vi "frontp_unregister_UI_user_events.vi"(8 "error in (no error)":errorcluster, 11 "front_panel in":refnum<class "front_panel.lvclass">) -> (0 "error out":errorcluster, 3 "front_panel out":refnum<class "front_panel.lvclass">)   [LabVIEW 2015, in "front_panel.lvclass"]
uses:
  front_panel.lvclass
  panel_class/panel.lvclass/panel.ctl
  front_panel.lvclass/front_panel.ctl
  panel_class/panel.lvclass
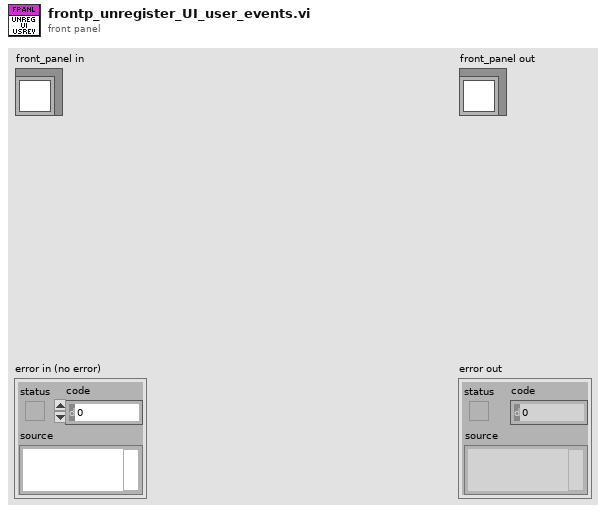
[diagram p1: front panel]
types:
  T1 = typedef "ui_registered_events.ctl" = cluster{"update_xy_graph":refnum<event-registration>, "update_graph":refnum<event-registration>, "update_chart":refnum<event-registration>, "update_map":refnum<event-registration>, "event_loop_stop":refnum<event-registration>, "keep_map":refnum<event-registration>}
  T2 = typedef "ui_user_events.ctl" = cluster{"update_xy_graph":refnum<user-event>, "update_graph":refnum<user-event>, "update_chart":refnum<user-event>, "update_map":refnum<user-event>, "event_loop_stop":refnum<user-event>, "keep_map":refnum<user-event>}
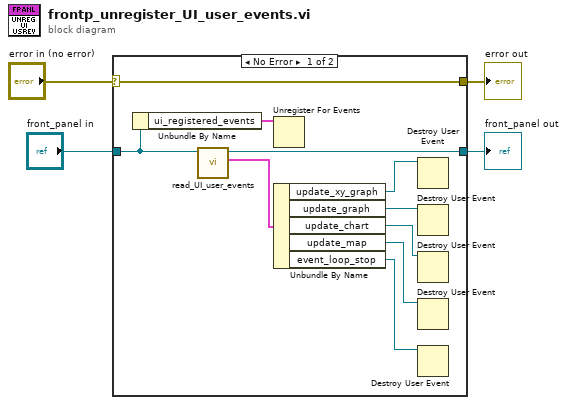
[diagram p0: block diagram]
diagram:
  n1 = case shown="No Error" "error in (no error)" {
    selector: "error in (no error)" -> [w14 w16]
    tunnel: [w14 w16] -> w3
    tunnel: [w5 w15] -> w1
    tunnel: "front_panel in" -> [w8 w15]
    frame No Error {
      n2 = Unbundle By Name(w8) -> ("ui_registered_events"=w7:T1)
      n3 = call "read_UI_user_events.vi"("panel in"=w8) -> ("ui_user_events"=w6:T2, "panel out"=w5:refnum<class "front_panel.lvclass">)  [unwired: 8 in, 1 out]
      n4 = Unregister For Events(event registration refnum=w7) -> ()  [unwired: 1 in, 1 out]
      n5 = Unbundle By Name(w6) -> ("update_xy_graph"=w13:refnum<user-event>, "update_graph"=w12:refnum<user-event>, "update_chart"=w11:refnum<user-event>, "update_map"=w10:refnum<user-event>, "event_loop_stop"=w9:refnum<user-event>)
      n6 = Destroy User Event(user event=w13) -> ()  [unwired: 1 in, 1 out]
      n7 = Destroy User Event(user event=w12) -> ()  [unwired: 1 in, 1 out]
      n8 = Destroy User Event(user event=w11) -> ()  [unwired: 1 in, 1 out]
      n9 = Destroy User Event(user event=w10) -> ()  [unwired: 1 in, 1 out]
      n10 = Destroy User Event(user event=w9) -> ()  [unwired: 1 in, 1 out]
    }
    frame Error {
    }
  }
  "error out" <- w3
  "front_panel out" <- w1
